vi "Info.vi"(8 "error in (no error)":errorcluster, 11 "Channel in":refnum<class "Channel.lvclass">) -> (0 "error out":errorcluster, 2 "Info":T1, 3 "Channel out":refnum<class "Channel.lvclass">)   [LabVIEW 2020, in "Vecto.lvlib" / "Channel.lvclass"]
uses:
  Channel.lvclass
  Channel Info.ctl
  Channel.lvclass/Channel.ctl
  Group/Group.lvclass
  C:/dev/lv20CE/relink/lv-vecto/Vecto/GroupAbstract/GroupAbstract.lvclass
  GroupAbstract/GroupAbstract.lvclass
  Vecto.lvlib
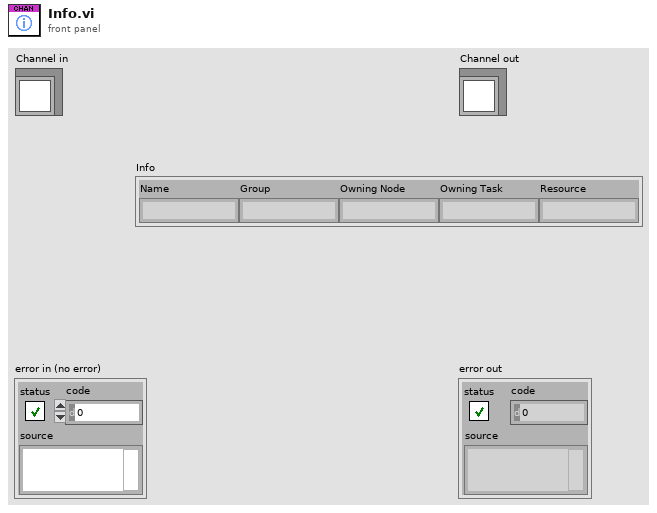
[diagram p1: front panel]
types:
  T1 = typedef "Vecto.lvlib/Channel Info.ctl" = cluster{"Name":string, "Group":string, "Owning Node":string, "Owning Task":string, "Resource":string}
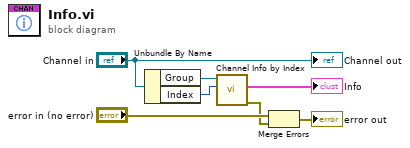
[diagram p0: block diagram]
diagram:
  n1 = Unbundle By Name("Channel in") -> ("Group"=w4:refnum<class "Group.lvclass">, "Index"=w2:i32)
  n2 = call "Channel Info by Index.vi"("Index"=w2, "GroupAbstract in"=w4) -> ("error out"=w3:errorcluster, "Channel Info"=→"Info":T1)  [unwired: 7 in, 1 out]
  n3 = Merge Errors("error in (no error)", w3) -> (→"error out":errorcluster)
  "Channel out" <- "Channel in"
